vi "renderVideoPage.vi"(8 "error in (no error)":errorcluster, 10 "VideoId":string, 11 "YoutuberDownloader in":refnum<class "YoutuberDownloader.lvclass">) -> (0 "error out":errorcluster, 3 "YoutuberDownloader out":refnum<class "YoutuberDownloader.lvclass">)   [LabVIEW 2017, in "YoutuberDownloader.lvclass"]
uses:
  YoutuberDownloader.lvclass
  YoutuberDownloader.lvclass/YoutuberDownloader.ctl
  Video Class/Video.lvclass/Video.ctl
  Globals/ConsoleOut.vi
  ThirdPartyYoutubeLib Class/ThirdPartyYoutubeLib.lvclass
  Video Class/Video.lvclass
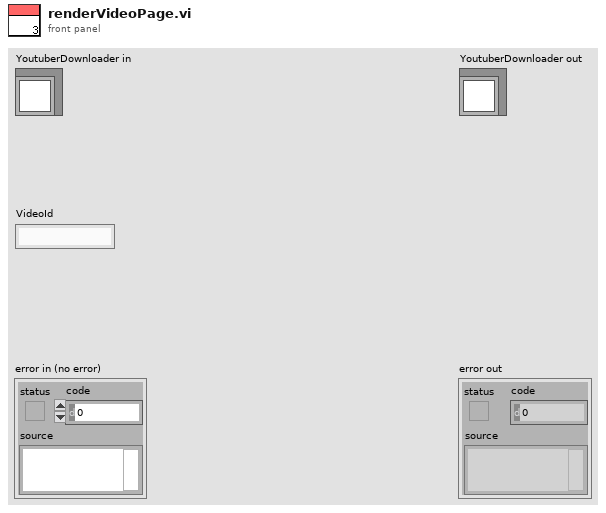
[diagram p1: front panel]
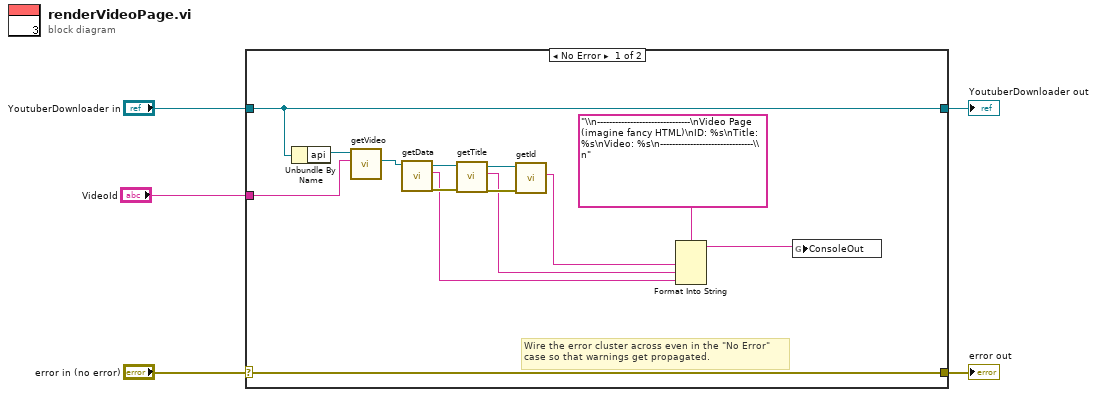
[diagram p0: block diagram]
diagram:
  n1 = case shown="No Error" "error in (no error)" {
    selector: "error in (no error)" -> [w19 w21]
    tunnel: [w19 w21] -> w4
    tunnel: [w18 w20] -> w2
    tunnel: "YoutuberDownloader in" -> [w18 w20]
    tunnel: "VideoId" -> [w16 _]
    frame No Error {
      # "Wire the error cluster across even in the \"No Error\"\ncase so that warnings get propagated."
      n2 = Unbundle By Name(w18) -> ("api"=w17:refnum<class "ThirdPartyYoutubeLib.lvclass">)
      n3 = call-dynamic "getVideo.vi"("Video Id"=w16, "ThirdPartyYoutubeLib in"=w17) -> ("Video"=w9:refnum<class "Video.lvclass">)  [unwired: 7 in, 2 out]
      n4 = call "getData.vi"("Video in"=w9) -> ("error out"=w12:errorcluster, "data"=w8:string, "Video out"=w13:refnum<class "Video.lvclass">)  [unwired: 8 in]
      n5 = call "getTitle.vi"("error in (no error)"=w12, "Video in"=w13) -> ("error out"=w10:errorcluster, "title"=w7:string, "Video out"=w11:refnum<class "Video.lvclass">)  [unwired: 7 in]
      n6 = call "getId.vi"("error in (no error)"=w10, "Video in"=w11) -> ("id"=w6:string)  [unwired: 7 in, 2 out]
      n7 = Format Into String(format string="\\n-------------------------------\nVideo Page (imagine fancy HTML)\nID: %s\nTitle: %s\nVideo: %s\n-------------------------------\\n", w6, w7, w8) -> (resulting string=w14:string)  [unwired: 2 in, 1 out]
      n8 = global write "ConsoleOut.vi" "ConsoleOut"(w14) -> ()
    }
    frame Error {
    }
  }
  "error out" <- w4
  "YoutuberDownloader out" <- w2
